vi "Fpga-FIXParser.vi"() -> ()   [LabVIEW 2020]
uses:
  Common/Fpga-FIX.Parse.States.ctl
  Common/Fpga-Field.Value.ctl
  <vilib>/Platform/TimedLoop/XDataNode/timing_clust.ctl
  <vilib>/Platform/TimedLoop/XDataNode/nitl_modes.ctl
  <vilib>/Platform/TimedLoop/XDataNode/wakeup.ctl
  <vilib>/rvi/Emulation/niFpgaSctlEmulationGetInTimedLoop.vi
  <vilib>/rvi/Emulation/niFpgaEmulationReportErrorSimple.vi
  <vilib>/rvi/Emulation/niFpgaGetClockAttributes.vi
  <vilib>/rvi/Emulation/niFpgaCriticalErrorInLSC.vi
  <vilib>/rvi/Emulation/niFpgaEmulationIsFPGAContextNoSignature.vi
  <vilib>/rvi/errors/niFpgaSetErrorForExecOnDevCompSimple.vi
  <vilib>/rvi/eio/common/nirviEmuReportErrorAndStop.vi
  <vilib>/rvi/DataTransferAndStorage/Container/Common/niFpgaContainerGetUniqueNameForEmu.vi
  <vilib>/rvi/FIFO/Fifo_Resource/nirvififoEmulationSetSize.vi
  <vilib>/rvi/FIFO/Fifo_Resource/nirviFifoEmulationQueueMgr.vi
  <instcachedir>/0/nirviFifoEmulationQueueMgr_E5CAEC123FF24DC58D834DCA3CDAA9B5.lvgen/nirviFifoEmulationQueueMgr_E5CAEC123FF24DC58D834DCA3CDAA9B5_002.vi
  <vilib>/Utility/error.llb/Clear Errors.vi
  <vilib>/rvi/FIFO/Fifo_Resource/nirvififoEmulationCreateLock.vi
  <vilib>/rvi/Emulation/niFpgaProcessEmulError.vi
  <vilib>/rvi/FIFO/Fifo_Resource/nirvififoEmulationObtainLock.vi
  <vilib>/rvi/FIFO/Fifo_Resource/nirvififoEmulationReleaseLock.vi
  <vilib>/rvi/occurrence/nirviWaitOnOccurrenceBase.vi
  <vilib>/rvi/errors/nirviReportUnexpectedCaseInternalError.vi
  <vilib>/rvi/errors/nirviReportUnexpectedCaseInternalError (U32).vi
  <instcachedir>/0/nirviFifoEmulationQueueMgr_E5CAEC123FF24DC58D834DCA3CDAA9B5.lvgen/nirviFifoEmulationQueueMgr_E5CAEC123FF24DC58D834DCA3CDAA9B5_012.vi
  <vilib>/rvi/FIFO/Fifo_Resource/nirvififoEmulationDetermineInputValidOut.vi
  <vilib>/Platform/TimedLoop/XDataNode/XDataNode.xnode
  <vilib>/rvi/DataTransferAndStorage/Container/XNode/niFpgaContainer.xnode
  <vilib>/rvi/FIFO/Fifo_Resource/nirvififoEmulationRead.vi
  <vilib>/rvi/FIFO/Fifo_Resource/nirvififoEmulationWrite.vi
  <vilib>/Platform/TimedLoop/XDataNode/XDNodeRunTimeDep.lvlib
panel:
  out "Valid":bool
  out "YYMMDD":u32
  out "Valid":bool
  out "FieldNum":u16
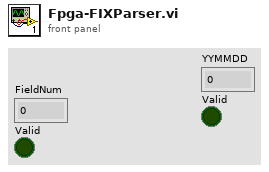
[diagram p1: front panel]
types:
  T1 = typedef "Fpga-Field.Value.ctl" = cluster{"Field.Num":u16, "Int.Value":u16, "Str.Value":u8[], "Date.Value":u64, "Str.Length":u8}
  T2 = typedef "Fpga-FIX.Parse.States.ctl" = enum16{"ReadNextField", "Read.Int.Value", "Read.Str.Value", "Read.Date.Value"}
  T3 = typedef "XDNodeRunTimeDep.lvlib/timing_clust.ctl" = cluster{"Expected End [f-1]":u64, "Actual End [f-1]":u64, "Finished Late? [f-1]":bool, "Expected End [i-1]":u64, "Actual End [i-1]":u64, "Finished Late? [i-1]":bool, "Expected Start [i]":u64, "Actual Start [i]":u64, "Expected Start [f]":u64, "Actual Start [f]":u64, "Source Name":string, "Structure Name":string, "Period":i64, "Deadline":i64, "Offset":i64, "Start":i64, "Priority":i32, "Timeout":i32, "Mode":T4, "Wakeup Reason":T5, "Error":errorcluster, "Source Type":string, "Secondary Source Type":string, "Global End Time":u64, "Global Start Time":u64, "Frame Duration":u64, "Iteration Duration":u64, "Assigned CPU":i32, "I/O Scan Engine Mode":u32}
  T4 = typedef "XDNodeRunTimeDep.lvlib/nitl_modes.ctl" = enum32{"No Change", "Process missed periods, maintain original phase", "Discard missed periods, maintain original phase", "Process missed periods, ignore original phase", "Discard missed periods, ignore original phase"}
  T5 = typedef "XDNodeRunTimeDep.lvlib/wakeup.ctl" = enum32{"Normal", "Aborted", "Asynchronous wakeup", "Timing source error", "Timed loop error", "Timeout"}
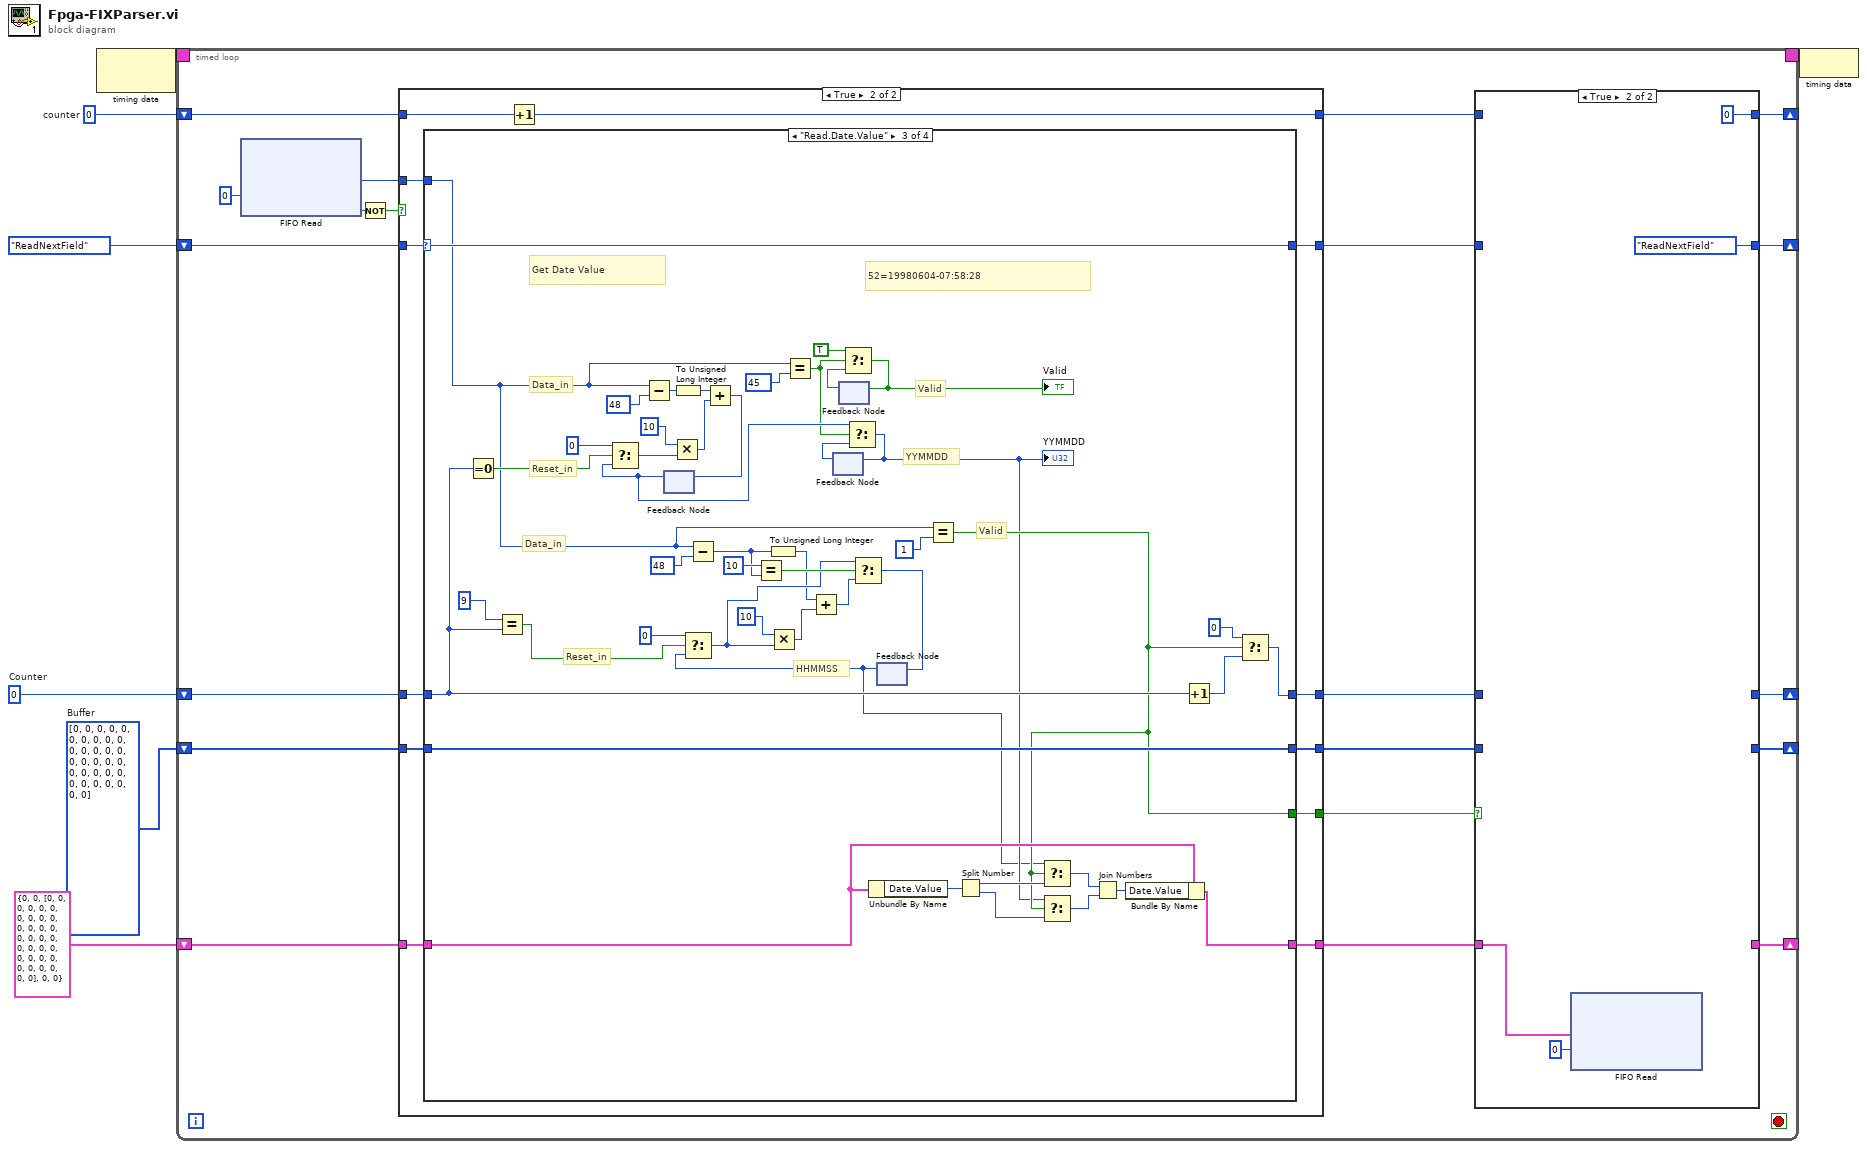
[diagram p0: block diagram]
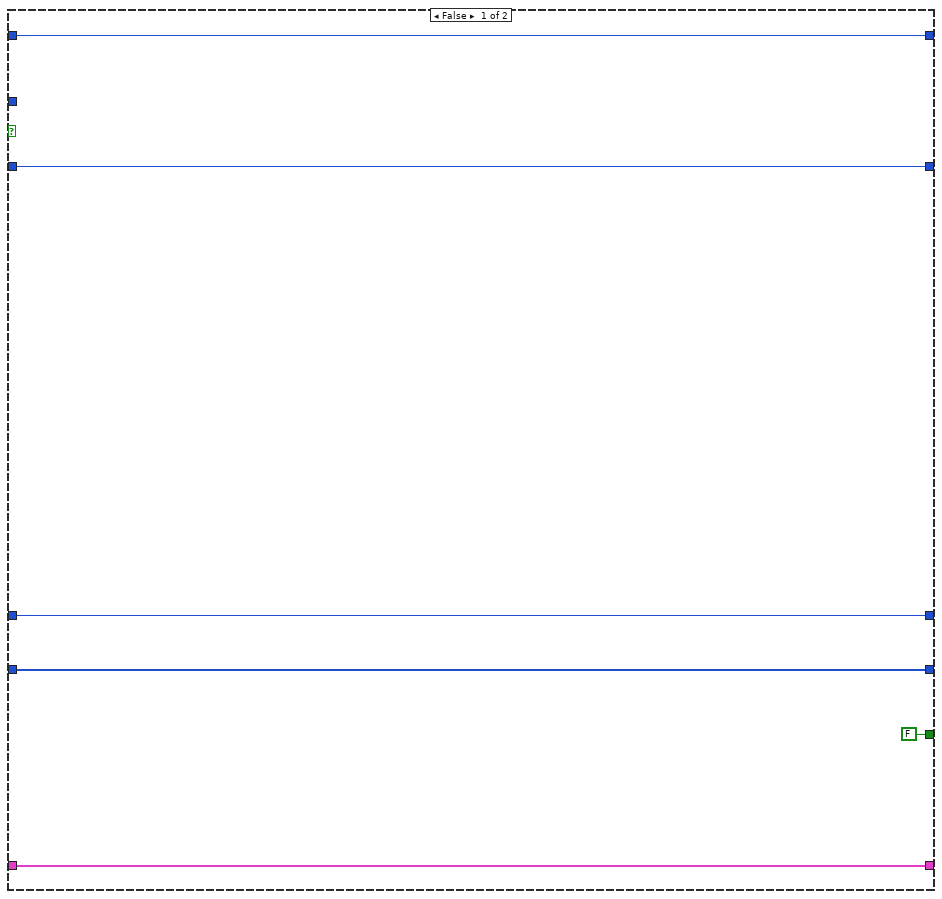
[diagram p3: hidden frame]
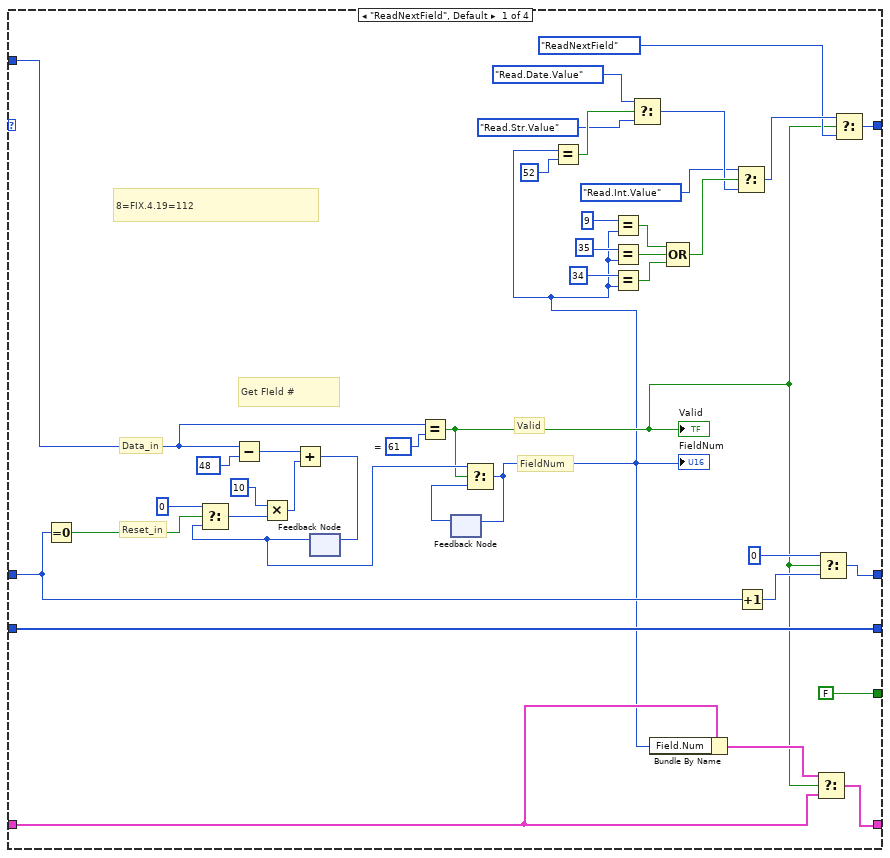
[diagram p4: hidden frame]
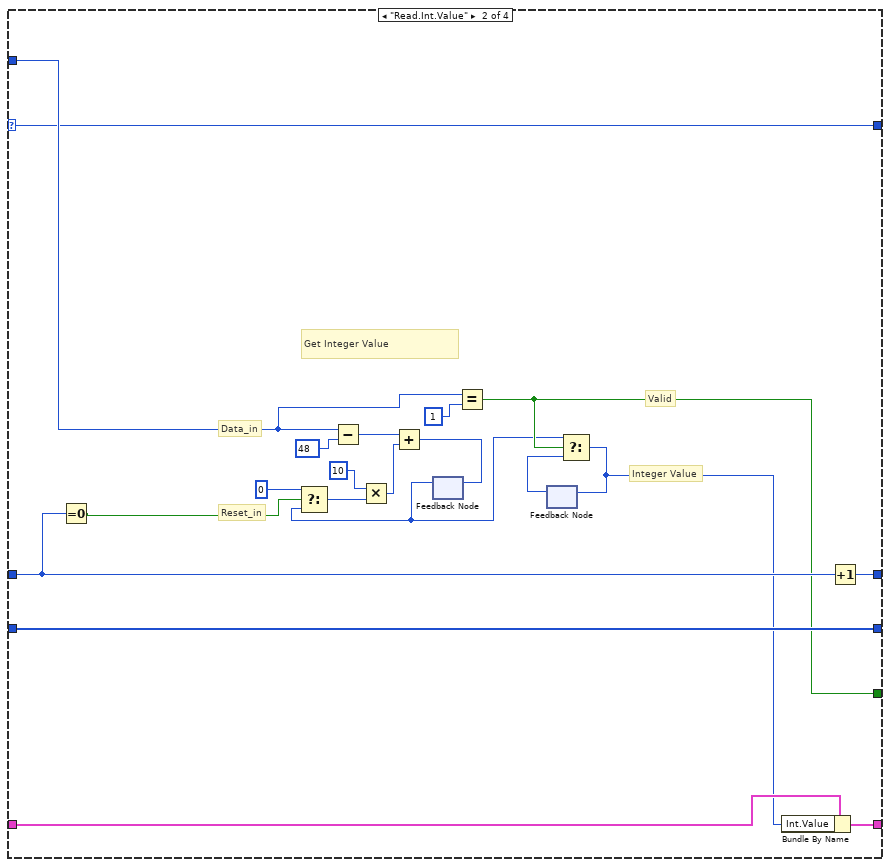
[diagram p5: hidden frame]
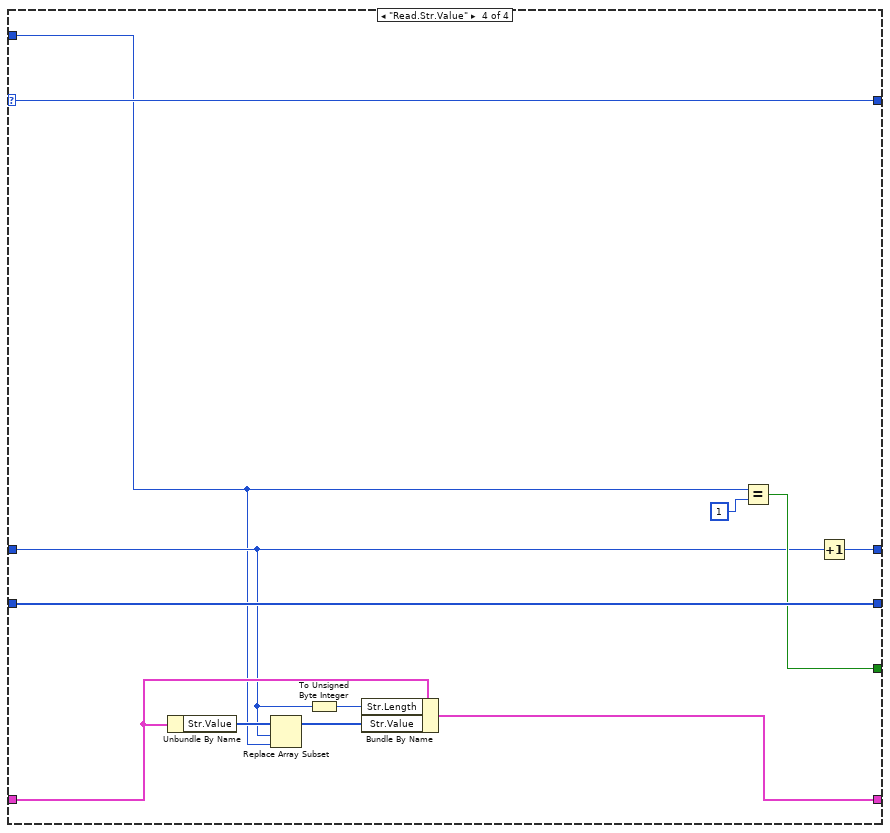
[diagram p6: hidden frame]
diagram:
  w2 = i16 0  # Counter
  w3 = u8[] [0, 0, 0, 0, 0, 0, 0, 0, 0, 0, 0, 0, 0, 0, 0, 0, 0, 0, 0, 0, 0, 0, 0, 0, 0, 0, 0, 0, 0, 0, 0, 0]  # Buffer
  w5 = u16 0  # counter
  n1 = node-c288() -> (w7:T3)  [unwired: 1 in]
  n2 = timed-loop {
    timing: w7 -> [_]
    timing-out: [_] -> w6
    shift-right: [w21] -> _
    shift-left: w5 -> [w23]
    shift-right: [w19] -> _
    shift-left: Fpga-FIX.Parse.States."ReadNextField" ("Side") -> [w20]
    shift-right: [w15] -> _
    shift-left: w3 -> [w16]
    shift-right: [w13] -> _
    shift-left: T1 {"Field.Num"=0, "Int.Value"=0, "Str.Value"=[0, 0, 0, 0, 0, 0, 0, 0, 0, 0, 0, 0, 0, 0, 0, 0, 0, 0, 0, 0, 0, 0, 0, 0, 0, 0, 0, 0, 0, 0, 0, 0], "Date.Value"=0, "Str.Length"=0} ("Field.Value.Pair") -> [w11]
    shift-right: [w9] -> _
    shift-left: w2 -> [w10]
    stop <- _ stop-if-true
    n3 = xnode ("FIFO Read")("Timeout"=0) -> ("Element"=w24:u8, "Timed Out?"=w26:bool)  [unwired: 1 in, 1 out]
    n4 = Not(x=w26) -> (.not. x?=w25:bool)
    n5 = case shown="True" w25 {
      tunnel: w24 -> [_ w51]
      tunnel: w23 -> [w42 w53]
      tunnel: [w42 w54] -> w22
      tunnel: w20 -> [w39 w52]
      tunnel: [w39 w50] -> w18
      tunnel: w10 -> [w40 w44]
      tunnel: [w40 w49] -> w17
      tunnel: w16 -> [w41 w48]
      tunnel: [w41 w47] -> w14
      tunnel: [w38 w46] -> w12
      tunnel: w11 -> [w38 w45]
      tunnel: [FALSE w43] -> w8
      frame False {
      }
      frame True {
        n6 = case shown="\"Read.Date.Value\"" w52 {
          selector: w52 -> [_ w101 w161 w173]
          tunnel: w51 -> [w86 w102 w121 w164]
          tunnel: [w93 w101 w161 w173] -> w50
          tunnel: w44 -> [w83 w104 w136 w165]
          tunnel: [w59 w112 w147 w169] -> w49
          tunnel: w48 -> [w92 w113 w160 w172]
          tunnel: [w92 w113 w160 w172] -> w47
          tunnel: [w61 w100 w152 w168] -> w46
          tunnel: w45 -> [w63 w99 w140 w167]
          tunnel: [FALSE w96 w116 w170] -> w43
          frame "ReadNextField", Default {
            w87 = u8 61  # =
            # "Valid"
            # "FieldNum"
            # "Reset_in"
            # "Data_in"
            # "Get FIeld #"
            # "8=FIX.4.19=112"
            n7 = Equal To 0?(x=w83) -> (x = 0?=w82:bool)
            n8 = Subtract(x=w86, y=u8 48) -> (x-y=w89:u8)
            n9 = feedback #1() -> (w81:u16)  [unwired: 1 in]
            n10 = Select(t=u16 0, s=w82, f=w81) -> (s? t:f=w80:u16)
            n11 = Multiply(x=u16 10 ("y"), y=w80) -> (x*y=w88:u16)
            n12 = Add(x=w89, y=w88) -> (x+y=w85:u16)
            n13 = feedback-in #1(w85) -> ()
            n14 = Equal?(x=w86, y=w87) -> (x = y?=w56:bool)
            "Valid" <- w56
            n15 = feedback #2() -> (w84:u16)  [unwired: 1 in]
            n16 = Select(t=w81, s=w56, f=w84) -> (s? t:f=w55:u16)
            "FieldNum" <- w55
            n17 = feedback-in #2(w55) -> ()
            n18 = Equal?(x=w55, y=u16 52 ("x")) -> (x = y?=w65:bool)
            n19 = Equal?(x=u16 9, y=w55) -> (x = y?=w74:bool)
            n20 = Equal?(x=u16 35, y=w55) -> (x = y?=w73:bool)
            n21 = Equal?(x=u16 34, y=w55) -> (x = y?=w72:bool)
            n22 = Select(t=Fpga-FIX.Parse.States."Read.Date.Value" ("Side"), s=w65, f=Fpga-FIX.Parse.States."Read.Str.Value" ("Side")) -> (s? t:f=w70:T2)
            n23 = Bundle By Name(cluster=w63, "Field.Num"=w55) -> (w62:T1)
            n24 = Compound Arithmetic op=OR(w74, w73, w72) -> (w71:bool)
            n25 = Select(t=Fpga-FIX.Parse.States."Read.Int.Value" ("Side"), s=w71, f=w70) -> (s? t:f=w69:T2)
            n26 = Increment(x=w83) -> (x+1=w57:i16)
            n27 = Select(t=w62, s=w56, f=w63) -> (s? t:f=w61:T1)
            n28 = Select(t=i16 0 ("Counter"), s=w56, f=w57) -> (s? t:f=w59:i16)
            n29 = Select(t=w69, s=w56, f=Fpga-FIX.Parse.States."ReadNextField" ("Side")) -> (s? t:f=w93:T2)
          }
          frame "Read.Int.Value" {
            # "Integer Value"
            # "Valid"
            # "Reset_in"
            # "Data_in"
            # "Get Integer Value"
            n30 = Equal To 0?(x=w104) -> (x = 0?=w103:bool)
            n31 = Subtract(x=w102, y=u8 48) -> (x-y=w108:u8)
            n32 = feedback #3() -> (w95:u16)  [unwired: 1 in]
            n33 = Select(t=u16 0, s=w103, f=w95) -> (s? t:f=w106:u16)
            n34 = Multiply(x=u16 10 ("y"), y=w106) -> (x*y=w107:u16)
            n35 = Add(x=w108, y=w107) -> (x+y=w98:u16)
            n36 = feedback-in #3(w98) -> ()
            n37 = Equal?(x=w102, y=u8 1 ("x")) -> (x = y?=w96:bool)
            n38 = feedback #4() -> (w97:u16)  [unwired: 1 in]
            n39 = Select(t=w95, s=w96, f=w97) -> (s? t:f=w94:u16)
            n40 = feedback-in #4(w94) -> ()
            n41 = Bundle By Name(cluster=w99, "Int.Value"=w94) -> (w100:T1)
            n42 = Increment(x=w104) -> (x+1=w112:i16)
          }
          frame "Read.Date.Value" {
            # "HHMMSS"
            # "Valid"
            # "YYMMDD"
            # "Valid"
            # "Reset_in"
            # "Data_in"
            # "52=19980604-07:58:28"
            # "Reset_in"
            # "Data_in"
            # "Get Date Value"
            n43 = Equal To 0?(x=w136) -> (x = 0?=w153:bool)
            n44 = Equal?(x=i16 9, y=w136) -> (x = y?=w141:bool)
            n45 = Subtract(x=w121, y=u8 48) -> (x-y=w135:u8)
            n46 = feedback #5() -> (w130:u32)  [unwired: 1 in]
            n47 = Select(t=u32 0, s=w153, f=w130) -> (s? t:f=w155:u32)
            n48 = Multiply(x=u32 10 ("y"), y=w155) -> (x*y=w156:u32)
            n49 = To Unsigned Long Integer(number=w135) -> (unsigned 32bit integer=w151:u32)
            n50 = Subtract(x=w121, y=u8 48) -> (x-y=w123:u8)
            n51 = Add(x=w151, y=w156) -> (x+y=w131:u32)
            n52 = feedback-in #5(w131) -> ()
            n53 = Equal?(x=u8 10, y=w123) -> (x = y?=w138:bool)
            n54 = To Unsigned Long Integer(number=w123) -> (unsigned 32bit integer=w122:u32)
            n55 = Equal?(x=w121, y=u8 45 ("x")) -> (x = y?=w128:bool)
            n56 = feedback #6() -> (w132:u32)  [unwired: 1 in]
            n57 = feedback #7() -> (w127:bool)  [unwired: 1 in]
            n58 = Select(t=TRUE, s=w128, f=w127) -> (s? t:f=w125:bool)
            "Valid" <- w125
            n59 = feedback-in #7(w125) -> ()
            n60 = Select(t=w130, s=w128, f=w132) -> (s? t:f=w115:u32)
            "YYMMDD" <- w115
            n61 = feedback-in #6(w115) -> ()
            n62 = Unbundle By Name(w140) -> ("Date.Value"=w149:u64)
            n63 = feedback #8() -> (w114:u32)  [unwired: 1 in]
            n64 = Select(t=u32 0, s=w141, f=w114) -> (s? t:f=w134:u32)
            n65 = Multiply(x=u32 10 ("y"), y=w134) -> (x*y=w143:u32)
            n66 = Add(x=w122, y=w143) -> (x+y=w133:u32)
            n67 = Select(t=w134, s=w138, f=w133) -> (s? t:f=w137:u32)
            n68 = feedback-in #8(w137) -> ()
            n69 = Equal?(x=w121, y=u8 1 ("x")) -> (x = y?=w116:bool)
            n70 = Split Number(x=w149) -> (hi(x)=w118:u32, lo(x)=w119:u32)
            n71 = Select(t=w114, s=w116, f=w118) -> (s? t:f=w117:u32)
            n72 = Select(t=w115, s=w116, f=w119) -> (s? t:f=w120:u32)
            n73 = Join Numbers(hi=w117, lo=w120) -> ((hi.lo)=w145:u64)
            n74 = Bundle By Name(cluster=w140, "Date.Value"=w145) -> (w152:T1)
            n75 = Increment(x=w136) -> (x+1=w146:i16)
            n76 = Select(t=i16 0 ("Counter"), s=w116, f=w146) -> (s? t:f=w147:i16)
          }
          frame "Read.Str.Value" {
            n77 = Unbundle By Name(w167) -> ("Str.Value"=w166:u8[])
            n78 = Replace Array Subset(array=w166, new element=w164, index=w165) -> (w163:u8[])
            n79 = To Unsigned Byte Integer(number=w165) -> (unsigned 8bit integer=w162:u8)
            n80 = Bundle By Name(cluster=w167, "Str.Length"=w162, "Str.Value"=w163) -> (w168:T1)
            n81 = Equal?(x=w164, y=u8 1 ("x")) -> (x = y?=w170:bool)
            n82 = Increment(x=w165) -> (x+1=w169:i16)
          }
        }
        n83 = Increment(x=w53) -> (x+1=w54:u16)
      }
    }
    n84 = case shown="True" w8 {
      tunnel: w22 -> [w32 _]
      tunnel: [w32 u16 0 ("counter")] -> w21
      tunnel: [w31 Fpga-FIX.Parse.States."ReadNextField" ("Side")] -> w19
      tunnel: w18 -> [w31 _]
      tunnel: [w30 _] -> w9
      tunnel: w17 -> [w30 _]
      tunnel: [w29 _] -> w15
      tunnel: w14 -> [w29 _]
      tunnel: [w28 _] -> w13
      tunnel: w12 -> [w28 w33]
      frame False {
      }
      frame True {
        n85 = xnode ("FIFO Read")("Element"=w33, "Timeout"=0) -> ()  [unwired: 1 in, 2 out]
      }
    }
  }
  n86 = node-c288(w6) -> ()
